vi "BlockTactic.vi"(8 "error in (no error)":errorcluster, 9 "Game in":refnum<class "Game.lvclass">, 10 "Robot":refnum<class "Robot.lvclass">, 11 "AttackerBlockTactic in":refnum<class "AttackerBlockTactic.lvclass">) -> (0 "error out":errorcluster, 2 "Robot out":refnum<class "Robot.lvclass">, 3 "AttackerBlockTactic out":refnum<class "AttackerBlockTactic.lvclass">)   [LabVIEW 2018, in "AttackerBlockTactic.lvclass"]
uses:
  AttackerBlockTactic.lvclass
  Game_class/Game.lvclass
  Robot_class/Robot.lvclass
  C:/Users/Rebeca/Documents/Rebeca/Roboime/SSL_AI - Carla/Tactic_class/Tactic.lvclass
  Tactic_class/Tactic.lvclass/Tactic.ctl
  States.ctl
  Skillbook_class/Skillbook.lvclass/Skillbook.ctl
  Game_class/Game.lvclass/Game.ctl
  Parameters_class/Parameters.lvclass/Parameters.ctl
  AttackerBlockTactic.lvclass/AttackerBlockTactic.ctl
  Game_class/Read Parameters.lvclass.vi
  Parameters_class/Read AttakingOurselves.vi
  Skillbook_class/Read AttackerBlockSkill.vi
  Tactic_class/Read Skillbook.vi
  Write States.vi
  Skillbook_class/Skillbook.lvclass
  Parameters_class/Parameters.lvclass
  AttackerBlockSkill_class/AttackerBlockSkill.lvclass
panel:
  out "x .or. y?":bool
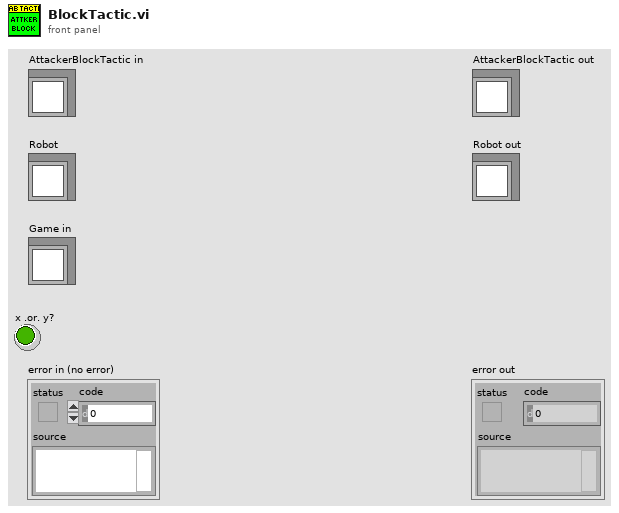
[diagram p1: front panel]
types:
  T1 = typedef "AttackerBlockTactic.lvclass/States.ctl" = enum16{"Block", "Exit"}
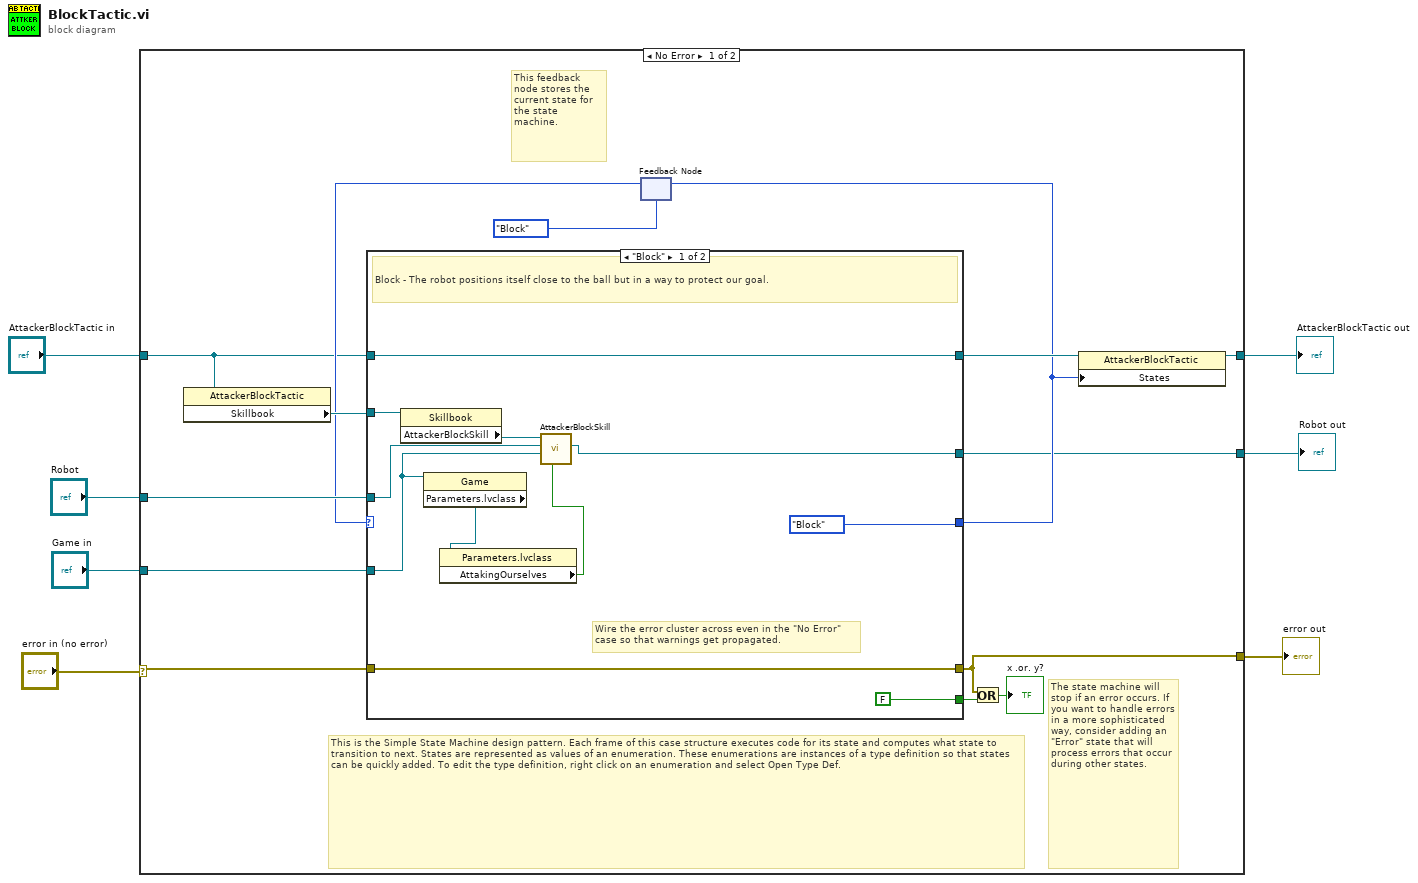
[diagram p0: block diagram]
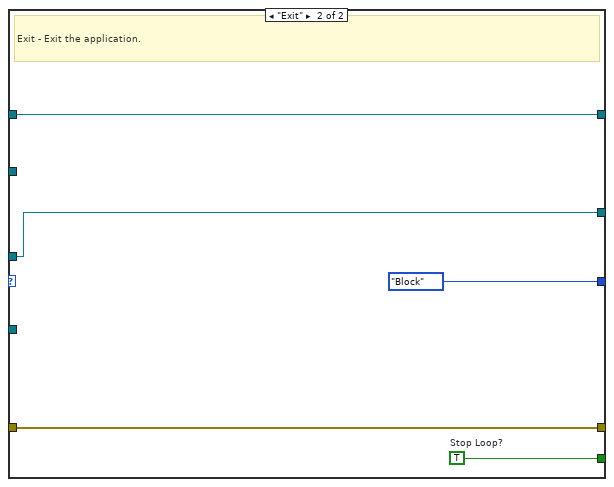
[diagram p2: hidden frame]
diagram:
  n1 = case shown="No Error" "error in (no error)" {
    selector: "error in (no error)" -> [w11 w40]
    tunnel: [w12 w40] -> w6
    tunnel: [w14 w39] -> w4
    tunnel: "AttackerBlockTactic in" -> [w8 w39]
    tunnel: "Robot" -> [w16 w38]
    tunnel: "Game in" -> [w15 _]
    tunnel: [w13 w38] -> w1
    frame No Error {
      # "The state machine will stop if an error occurs. If you want to handle errors in a more sophisticated way, consider adding an \"Error\" state that will process errors that occur during other states."
      # "This feedback node stores the current state for the state machine."
      # "This is the Simple State Machine design pattern. Each frame of this case structure executes code for its state and computes what state to transition to next. States are represented as values of an enumeration. These enumerations are instances of a type definition so that states can be quickly added. To edit the type definition, right click on an enumeration and select Open Type Def."
      # "Wire the error cluster across even in the \"No Error\"\ncase so that warnings get propagated."
      n2 = property class="AttackerBlockTactic"(reference=w8) -> ("Skillbook"=w19:refnum<class "Skillbook.lvclass">)  [unwired: 1 in, 2 out]
      n3 = feedback #1(States."Block" ("States")) -> (w9:T1)
      n4 = case shown="\"Block\"" w9 {
        tunnel: [States."Block" ("States") States."Block" ("States")] -> w17
        tunnel: [FALSE ("Stop Loop?") w37] -> w21
        tunnel: w11 -> [w31 w36]
        tunnel: [w31 w36] -> w12
        tunnel: w19 -> [w30 _]
        tunnel: w16 -> [w26 w35]
        tunnel: [w25 w35] -> w13
        tunnel: [w29 w34] -> w18
        tunnel: w8 -> [w29 w34]
        tunnel: w15 -> [w24 _]
        frame "Block" {
          # "Block - The robot positions itself close to the ball but in a way to protect our goal."
          n5 = property class="Skillbook"(reference=w30) -> ("AttackerBlockSkill"=w27:refnum<class "AttackerBlockSkill.lvclass">)  [unwired: 1 in, 2 out]
          n6 = property class="Game"(reference=w24) -> ("Parameters.lvclass"=w23:refnum<class "Parameters.lvclass">)  [unwired: 1 in, 2 out]
          n7 = property class="Parameters.lvclass"(reference=w23) -> ("AttakingOurselves"=w22:bool)  [unwired: 1 in, 2 out]
          n8 = call-dynamic "AttackerBlockSkill.vi"("AttackOurselves"=w22, "Game"=w24, "Robot"=w26, "AttackerBlockSkill in"=w27) -> ("Robot out"=w25:refnum<class "Robot.lvclass">)  [unwired: 5 in, 2 out]
        }
        frame "Exit" {
          w37 = TRUE  # Stop Loop?
          # "Exit - Exit the application."
        }
      }
      n9 = feedback-in #1(w17) -> ()
      n10 = Or(x=w12, y=w21) -> (x .or. y?=→"x .or. y?":bool)
      n11 = property class="AttackerBlockTactic"(reference=w18, "States"=w17) -> (reference out=w14:refnum<class "AttackerBlockTactic.lvclass">)  [unwired: 1 in, 1 out]
    }
    frame Error {
    }
  }
  "error out" <- w6
  "AttackerBlockTactic out" <- w4
  "Robot out" <- w1
